vi "file header.vi"(9 "channel strings":string[](array[string]), 11 "refnum":refnum<file>) -> (3 "dup refnum":refnum<file>)   [LabVIEW 2012]
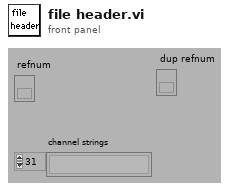
[diagram p1: front panel]
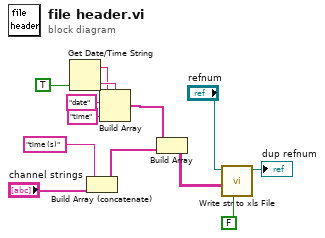
[diagram p0: block diagram]
diagram:
  n1 = Get Date/Time String(want seconds? (F)=TRUE) -> (date string=w10:string, time string=w13:string)  [unwired: 2 in]
  n2 = Build Array (concatenate)("time (s)", "channel strings") -> (w4:string[])
  n3 = Build Array("date", w10, "time", w13) -> (w5:string[])
  n4 = Build Array(w5, w4) -> (w6:string[][])
  n5 = call "Write str to xls File.vi"("transpose? (no:F)"=FALSE, "2D data"=w6, "refnum"="refnum") -> ("dup refnum"=→"dup refnum":refnum<file>)  [unwired: 7 in, 1 out]
